vi "Emerson 5700 Units.vi"(8 "Error In":errorcluster, 11 "Emerson Flow Meter Data Input":T1) -> (0 "Error Out":errorcluster, 1 "Basic Units":string[](array[string]), 2 "Units with Mean, STD, ect":string[](array[string]), 3 "Emerson Flow Meter Data Output":T1)   [LabVIEW 2016]
uses:
  Type Definitions/Emerson 5700 Data.ctl
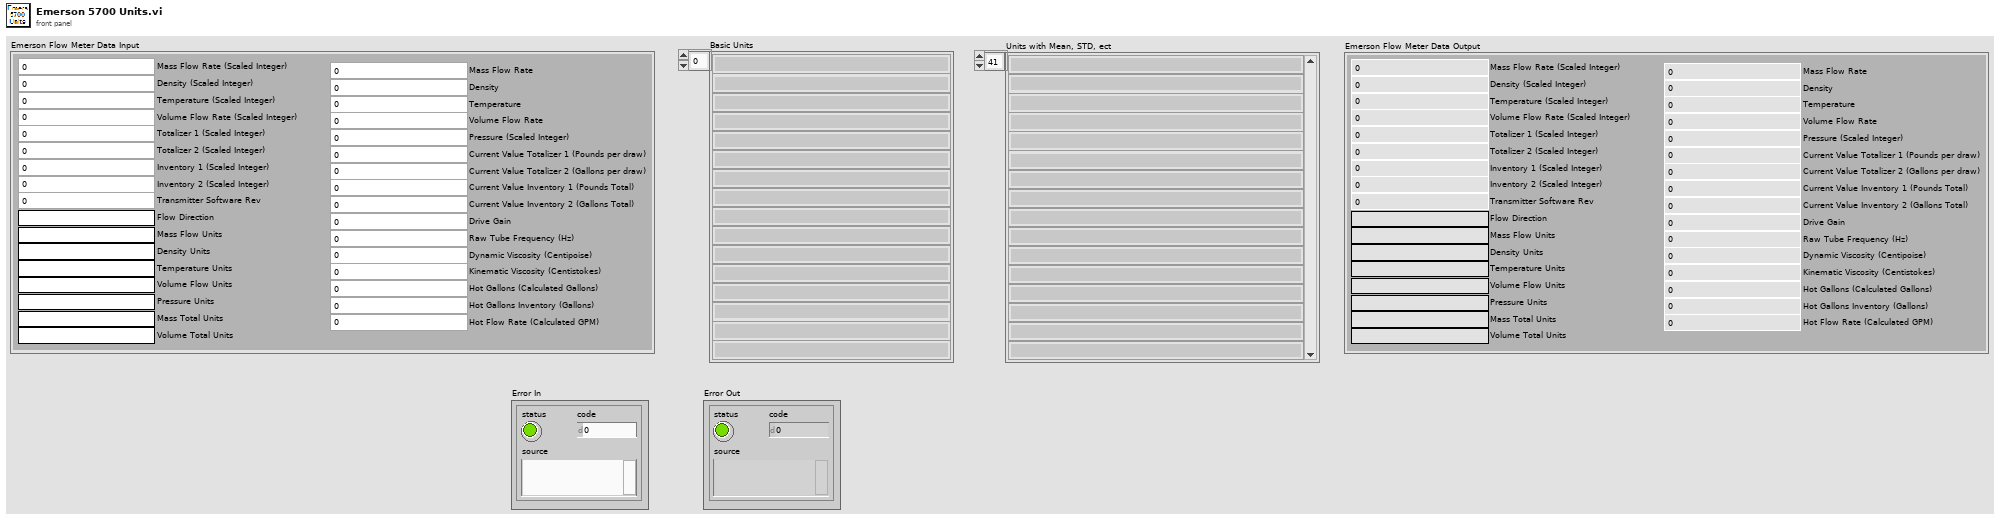
[diagram p1: front panel]
types:
  T1 = typedef "Emerson 5700 Data.ctl" = cluster{"Mass Flow Rate (Scaled Integer)":u16, "Density (Scaled Integer)":u16, "Temperature (Scaled Integer)":u16, "Volume Flow Rate (Scaled Integer)":u16, "Totalizer 1 (Scaled Integer)":u16, "Totalizer 2 (Scaled Integer)":u16, "Transmitter Software Rev":u16, "Flow Direction":string, "Mass Flow Units":string, "Density Units":string, "Temperature Units":string, "Volume Flow Units":string, "Pressure Units":string, "Mass Total Units":string, "Volume Total Units":string, "Inventory 1 (Scaled Integer)":u16, "Inventory 2 (Scaled Integer)":u16, "Mass Flow Rate":dbl, "Density":dbl, "Temperature":dbl, "Volume Flow Rate":dbl, "Pressure (Scaled Integer)":u16, "Current Value Totalizer 1 (Pounds per draw)":dbl, "Current Value Totalizer 2 (Gallons per draw)":dbl, "Current Value Inventory 1 (Pounds Total)":dbl, "Current Value Inventory 2 (Gallons Total)":dbl, "Drive Gain":dbl, "Raw Tube Frequency (Hz)":dbl, "Dynamic Viscosity (Centipoise)":dbl, "Kinematic Viscosity (Centistokes)":dbl, "Hot Gallons (Calculated Gallons)":dbl, "Hot Flow Rate (Calculated GPM)":dbl, "Hot Gallons Inventory (Gallons)":dbl}
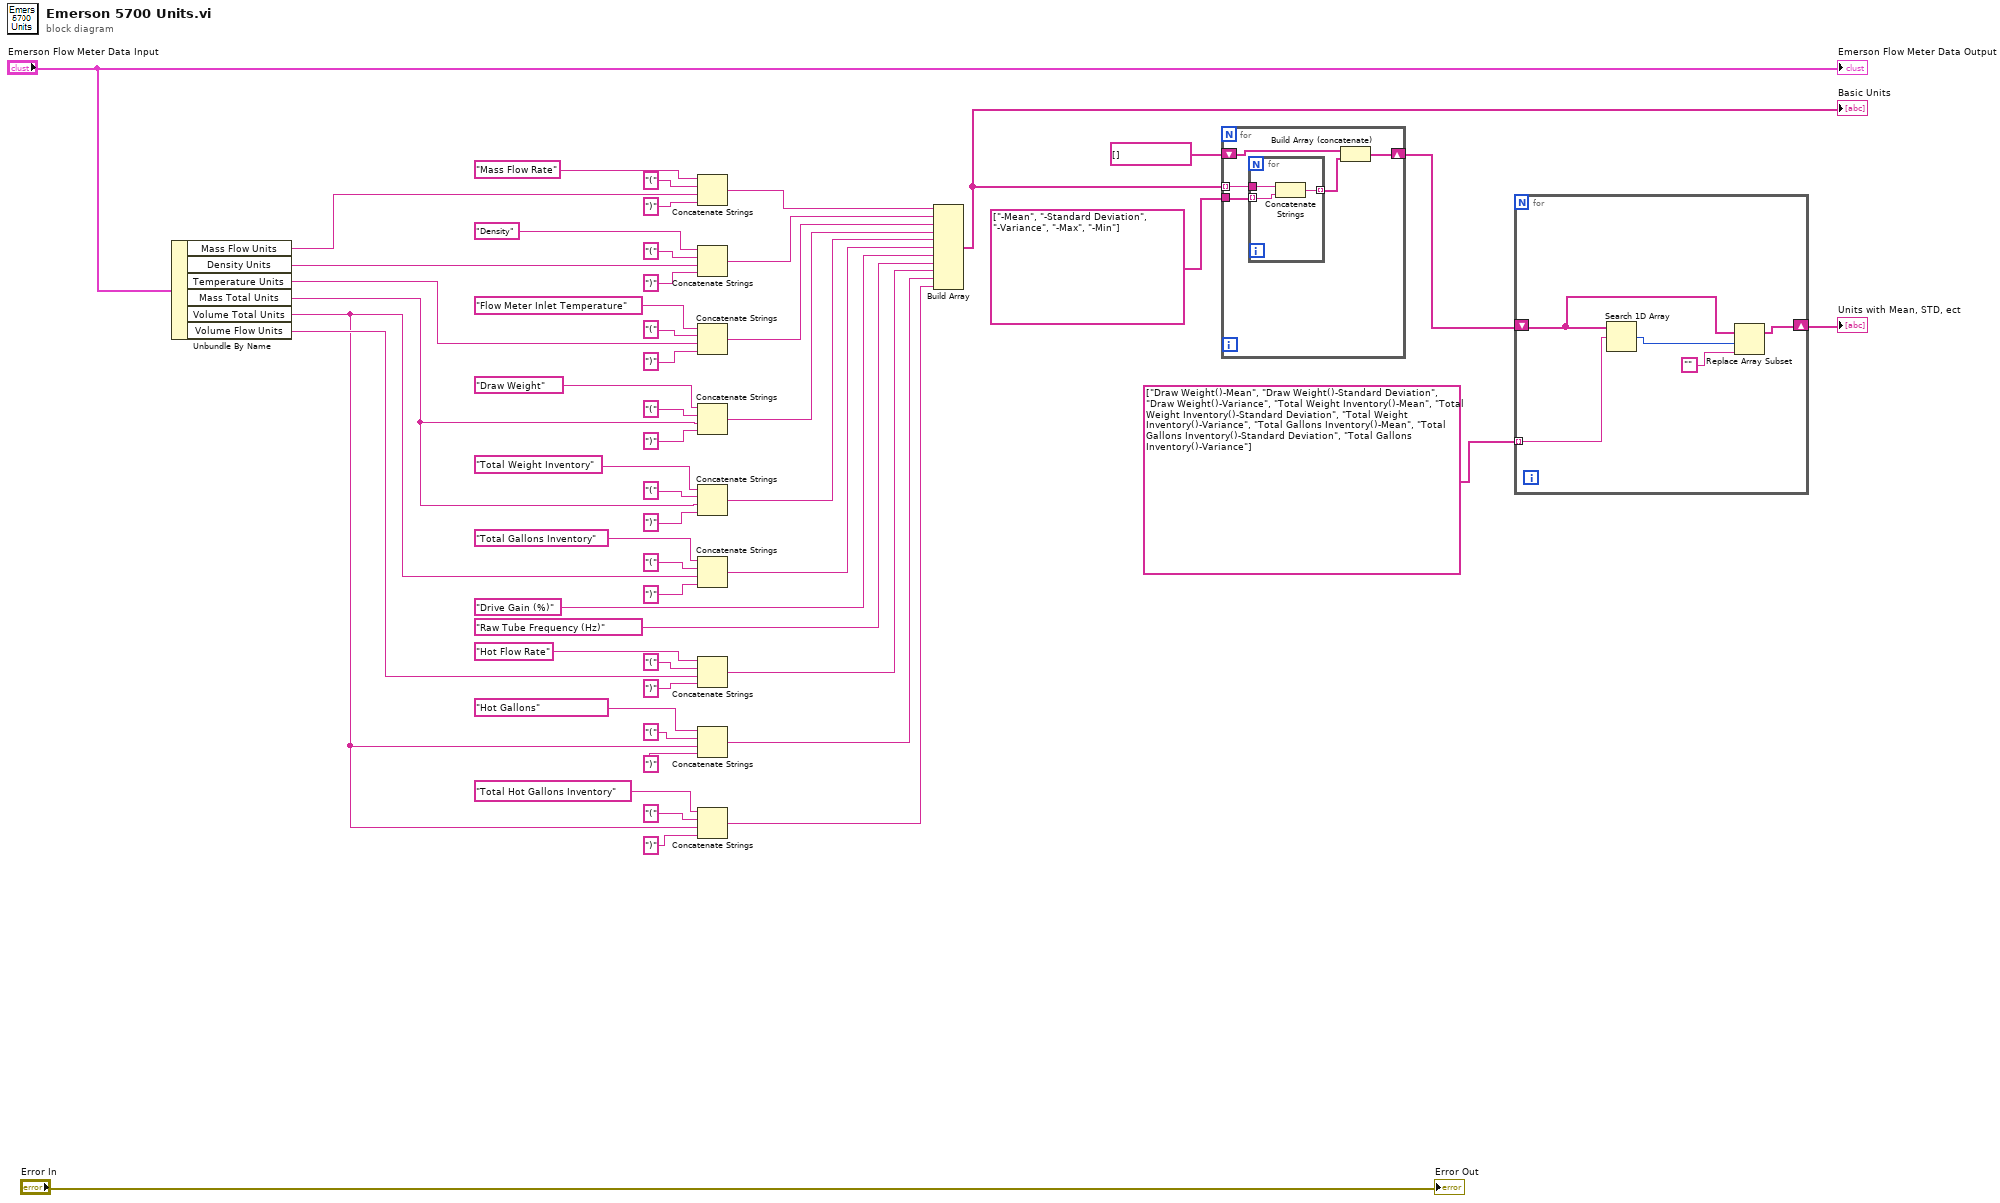
[diagram p0: block diagram]
diagram:
  n1 = Unbundle By Name("Emerson Flow Meter Data Input") -> ("Mass Flow Units"=w49:string, "Density Units"=w50:string, "Temperature Units"=w51:string, "Mass Total Units"=w52:string, "Volume Total Units"=w4:string, "Volume Flow Units"=w5:string)
  n2 = Concatenate Strings("Mass Flow Rate", "(" ("string"), w49, ")" ("string")) -> (w40:string)
  n3 = Concatenate Strings("Density", "(" ("string"), w50, ")" ("string")) -> (w41:string)
  n4 = Concatenate Strings("Flow Meter Inlet Temperature", "(" ("string"), w51, ")" ("string")) -> (w42:string)
  n5 = Concatenate Strings("Draw Weight", "(" ("string"), w52, ")" ("string")) -> (w43:string)
  n6 = Concatenate Strings("Total Weight Inventory", "(" ("string"), w52, ")" ("string")) -> (w44:string)
  n7 = Concatenate Strings("Total Gallons Inventory", "(" ("string"), w4, ")" ("string")) -> (w45:string)
  n8 = Concatenate Strings("Hot Flow Rate", "(" ("string"), w5, ")" ("string")) -> (w3:string)
  n9 = Concatenate Strings("Hot Gallons", "(" ("string"), w4, ")" ("string")) -> (w2:string)
  n10 = Concatenate Strings("Total Hot Gallons Inventory", "(" ("string"), w4, ")" ("string")) -> (w1:string)
  n11 = Build Array(w40, w41, w42, w43, w44, w45, "Drive Gain (%)", "Raw Tube Frequency (Hz)", w3, w2, w1) -> (w21:string[])
  "Basic Units" <- w21
  n12 = for {
    tunnel: w21 -> [w57] mode=indexing
    tunnel: string[] ["-Mean", "-Standard Deviation", "-Variance", "-Max", "-Min"] -> [w56]
    shift-right: [w53] -> w17
    shift-left: string[] [] -> [w55]
    n13 = for {
      tunnel: w57 -> [w60]
      tunnel: w56 -> [w59] mode=indexing
      tunnel: [w58] -> w54 mode=indexing
      n14 = Concatenate Strings(w60, w59) -> (w58:string)
    }
    n15 = Build Array (concatenate)(w55, w54) -> (w53:string[])
  }
  n16 = for {
    tunnel: string[] ["Draw Weight()-Mean", "Draw Weight()-Standard Deviation", "Draw Weight()-Variance", "Total Weight Inventory()-Mean", "Total Weight Inventory()-Standard Deviation", "Total Weight Inventory()-Variance", "Total Gallons Inventory()-Mean", "Total Gallons Inventory()-Standard Deviation", "Total Gallons Inventory()-Variance"] -> [w65] mode=indexing
    shift-right: [w61] -> w15
    shift-left: w17 -> [w64]
    n17 = Search 1D Array(1D array=w64, element=w65) -> (index of element=w63:i32)  [unwired: 1 in]
    n18 = Replace Array Subset(array=w64, new element="", index=w63) -> (w61:string[])
  }
  "Units with Mean, STD, ect" <- w15
  "Error Out" <- "Error In"
  "Emerson Flow Meter Data Output" <- "Emerson Flow Meter Data Input"
